vi "Set Plot Color (WDTWFGraph).vi"(8 "error in (no error)":errorcluster, 11 "WFGraph (WDT) in":refnum<vi>) -> (0 "error out":errorcluster)   [LabVIEW 2019, in "Instrument.Lockin.lvlib" / "Instrument UI.Lockin.lvclass"]
uses:
  Instrument UI.Lockin.lvclass
  <vilib>/PRIrvin/Graph Utilities/graph_utilities.lvclass
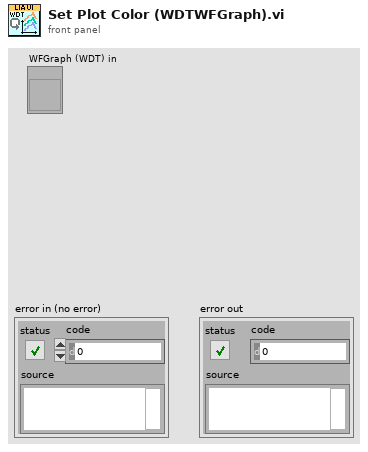
[diagram p1: front panel]
types:
  T1 = enum16{"CET-C1", "CET-C1s", "CET-C2", "CET-C2s", "CET-C3", "CET-C3s", "CET-C4", "CET-C4s", "CET-C5", "CET-C5s", "CET-C6", "CET-C6s", "CET-C7", "CET-C7s", "CET-CBC1", "CET-CBC2", "CET-CBD1", "CET-CBL1", "CET-CBL2", "CET-D01", "CET-D01A", "CET-D02", "CET-D03", "CET-D04", "CET-D06", "CET-D07", "CET-D08", "CET-D09", "CET-D10", "CET-D11", "CET-D12", "CET-D13", "CET-I1", "CET-I2", "CET-I3", "CET-L01", "CET-L02", "CET-L03", "CET-L04", "CET-L05", "CET-L06", "CET-L07", "CET-L08", "CET-L09", "CET-L10", "CET-L11", "CET-L12", "CET-L13", "CET-L14", "CET-L15", "CET-L16", "CET-L17", "CET-L18", "CET-L19", "CET-L20", "CET-R1", "CET-R2", "CET-R3", "CET-R4"}
  T2 = enum16{"Inferno", "Kindlmann", "Plasma", "Viridis", "LevyLab2010", "ColorCET...", "Custom..."}
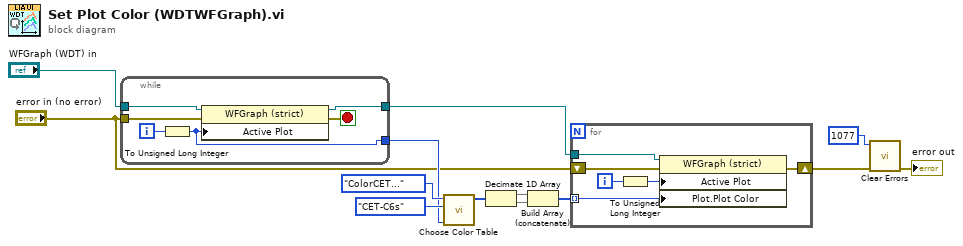
[diagram p0: block diagram]
diagram:
  n1 = while {
    tunnel: "WFGraph (WDT) in" -> [w19]
    tunnel: [w16] -> w3
    tunnel: [w15] -> w4
    tunnel: "error in (no error)" -> [w14]
    i -> [w18]
    stop <- w17 stop-if-true
    n2 = To Unsigned Long Integer(number=w18) -> (unsigned 32bit integer=w16:u32)
    n3 = property on="Property Node" class="WFGraph (strict)"(reference=w19, error in=w14, "Active Plot"=w16) -> (reference out=w15:refnum<vi>, error out=w17:errorcluster)
  }
  n4 = call <vilib>:"Choose Color Table.vi"("Size (256)"=w3, "ColorCET"=T1."CET-C6s", "Color Map"=T2."ColorCET...") -> ("Color Table"=w7:u32[])  [unwired: 5 in, 3 out]
  n5 = Decimate 1D Array(w7) -> (w11:u32[], w10:u32[])
  n6 = Build Array (concatenate)(w11, w10) -> (w2:u32[])
  n7 = for {
    tunnel: w2 -> [w24] mode=indexing
    tunnel: w4 -> [w22]
    shift-right: [w23] -> w6
    shift-left: "error in (no error)" -> [w25]
    i -> [w20]
    n8 = To Unsigned Long Integer(number=w20) -> (unsigned 32bit integer=w21:u32)
    n9 = property on="Property Node" class="WFGraph (strict)"(reference=w22, error in=w25, "Active Plot"=w21, "Plot.Plot Color"=w24) -> (error out=w23:errorcluster)  [unwired: 1 out]
  }
  n10 = call <vilib>:"Clear Errors.vi"("error in (no error)"=w6, "specific error code to clear (0: all)"=1077) -> ("error out"=→"error out":errorcluster)  [unwired: 4 in, 1 out]
